vi "DOE Software Model Type.vi"(8 "error in (no error)":errorcluster) -> (0 "error out":errorcluster, 3 "Software Model":T1)   [LabVIEW 2014]
doc: "There are several different types of software architecture. This will allow for the correct VI to be loaded into the main program at runtime"
uses:
  Type Definitions/DOE Software Model Type.ctl
  Utility/Custom Pallet Controls/Custom Pallet Forward.ctl
panel:
  out "Front Program Name 2":string="This appies to the following:\n1. Appliance.NET\n2. Laundry Tool\n3. Aquarium\n4. Ect"
  in  "File Setup OK":T2
  in  "Model Type":T1
  out "Front Program Name":string="Integrate External Software"
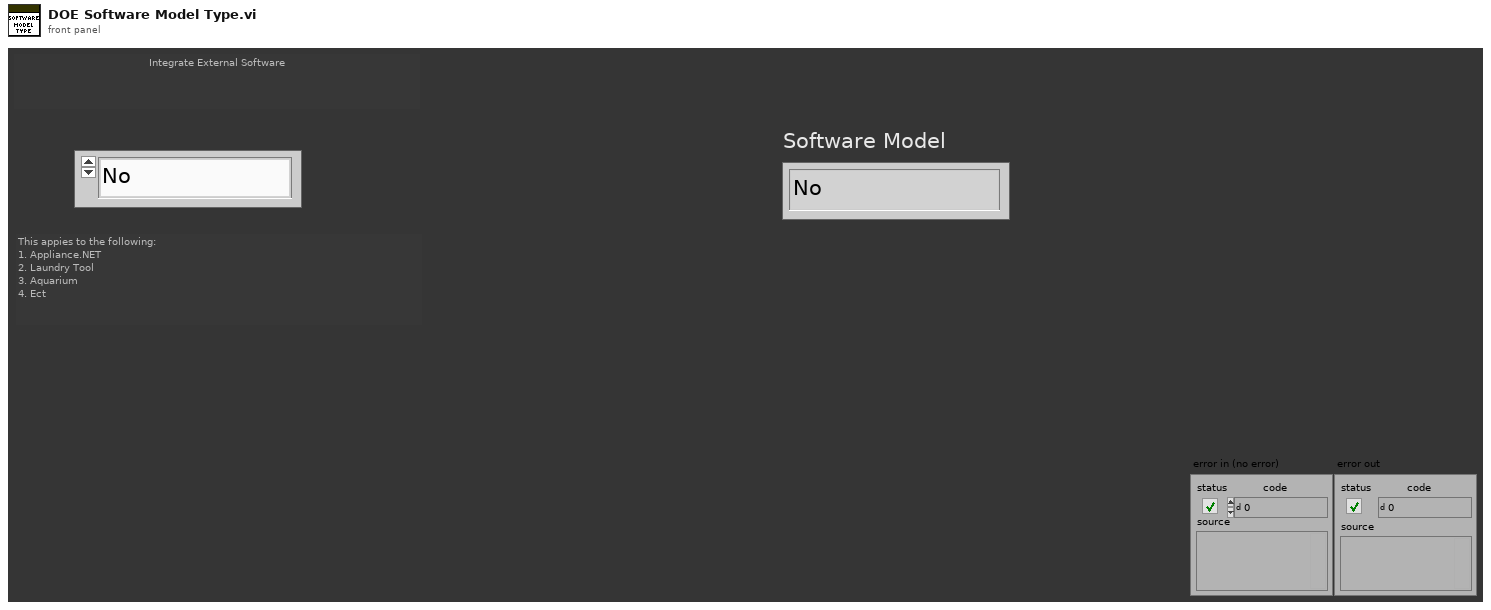
[diagram p1: front panel]
types:
  T1 = typedef "DOE Software Model Type.ctl" = enum16{"No", "Yes"}
  T2 = typedef "Custom Pallet Forward.ctl" = bool
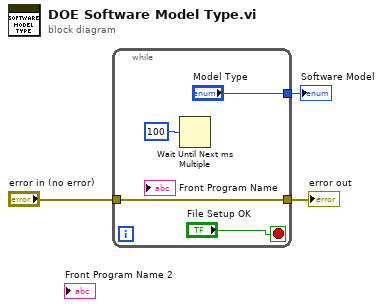
[diagram p0: block diagram]
diagram:
  n1 = while {
    tunnel: ["Model Type"] -> w1
    tunnel: "error in (no error)" -> [w4]
    tunnel: [w4] -> w2
    stop <- "File Setup OK" stop-if-true
    n2 = Wait Until Next ms Multiple(millisecond multiple=u32 100) -> ()  [unwired: 1 out]
  }
  "error out" <- w2
  "Software Model" <- w1
